vi "NI 5772 (AC) - TIS Mode Enabled (Host)_Independent.vi"() -> ()   [LabVIEW 2020]
doc: "Example Description:\nThis example demonstrates how to enable Time Interleaved Sampling with the NI 5772 adapter module to achieve a sampling rate of 1.6GS/s. This example continuously acquires records of analog input data from the NI 5772 adapter module. It allows you to select an AI channel, trigger type, and record size. This VI must be compiled before it is run. \n\nVI Configuration:\nThis example uses the NI PXI-7952R as the FPGA target by default. If you are using another FPGA target, complete the following steps to configure the host VI to use a VI configured for your FPGA target:\n1. On the block diagram, right-click the Open FPGA VI Reference (NI PXI-7952R) function and select Configure Open FPGA VI Reference.\n2. Browse for a new target by clicking the Browse Project button in the Open VI section.\n3. Select the VI under the target that matches your device. Click OK to select this VI.\n4. Click OK to exit the dialog box and to apply the new selection to the FPGA VI.\n5. Save the VI.\n\nRunning the VI:\n1. Select a RIO Resource that corresponds to the FPGA device configured above.\n2. Clock Configuration: Select the desired clock source for the adapter module.\nAnalog Input: Configure the AI Channel, Record Size, and Trigger Type controls. If you are using the analog trigger type, configure the Trigger Level (V) control.\n3. Click the run arrow to run the VI.\n4. If the Trigger Type is set to Software, click the Software Trigger button to acquire a single record of data. If the Trigger Type is set to Data Edge, a record of data is acquired each time the input signal rises above the trigger level.\n\nThe Record Size, Trigger Type, and Trigger Level (V) controls can all be configured while the VI is running. \n\nNote: The AI Channel control must be configured before the VI is run.\n\nExecution Steps:s\n1. Open a session to the FPGA VI and run the VI.\n2. Wait for the adapter module to load its default configuration.\n3. Configure the NI 5772 for Time Interleaved Sampling (TIS)\n4. The Trigger type and record size for a single record acquisition are configured.\n5. Based on the trigger type, either wait for the software trigger Boolean to assert or configure the desired trigger level and arm the trigger.\n6. After the trigger is armed, a single record of data is acquired and read.\n7. Stop the VI when the stop button is pressed or when an error has occurred. \n8. Close the FPGA VI reference and display any errors."
uses:
  <vilib>/userdefined/High Color/nirio_resource_hc.ctl
  Controls/TIS Mode.ctl
  Controls/FPGA VI Reference.ctl
  <vilib>/FPGAPlugInAG/PXIe-7962R/niLvFpga_Open_PXIe-7962R.vi
  <vilib>/rvi/interface/common/dynamic/niFpgaDynamicAddResources.vi
  <vilib>/Utility/error.llb/Error Cluster From Error Code.vi
  <vilib>/rvi/errors/niLvFpgaAdjustHostInterfaceError.vi
  <vilib>/FPGAPlugInAG/Dynamic/niLvFpga_Close_Dynamic.vi
  <vilib>/rvi/interface/nirviOpenFPGA/nirviOpenFPGA.xnode
  FPGA Bitfiles/acoustoxv3_FPGATarget_NI5772(AC)Digiti_U3W57aODG7w.lvbitx
  <vilib>/rvi/interface/nirviReadWriteControl/nirviReadWriteControl.xnode
  <vilib>/rvi/interface/nirviMethod/nirviMethod.xnode
  <vilib>/rvi/interface/nirviCloseFPGA/nirviCloseFPGA.xnode
  NiFpgaLv.dll
  <vilib>/rvi/interface/Simulation/niFpgaSimulationCallBeginRW.vi
  <vilib>/FPGAPlugInAG/Dynamic/niLvFpga_ReadFifo_Dynamic.vi
  <vilib>/rvi/errors/niLvFpgaMergeErrorWithErrorCode.vi
panel:
  in  "TrigIn_Sim":bool
  in  "TIS Mode":T1=3 items=["TIS Mode (CH0 Only)"=1, "TIS Mode (CH1 Only)"=2, "Dual TIS Mode (CH0 and CH1)"=3]
  out "TIS Configured?":bool
  out "Analog Input":waveform(ext)(graph)={"t0"=timestamp(0 s since 1904-01-01), "dt"=1.25e-09, "Y"=array[2048 elements]} caption="Acquired Waveform"
  out "error out":errorcluster
  in  "stop":bool
  in  "Trigger Level (V)":dbl
  in  "Software Trigger":bool=TRUE
  in  "Record Size":u16=1024
  in  "Trigger Type":enum8{"Software", "Data Edge"}(ring)
  in  "RIO Resource":T2="RIO0"
  out "Configured?":bool
  # "Resource Configuration"
  # "AI Configuration"
  # "For instructions, select Help>>Show Context Help and move the cursor over the VI icon to display help for this VI."
  # "Interleaved Configuration"
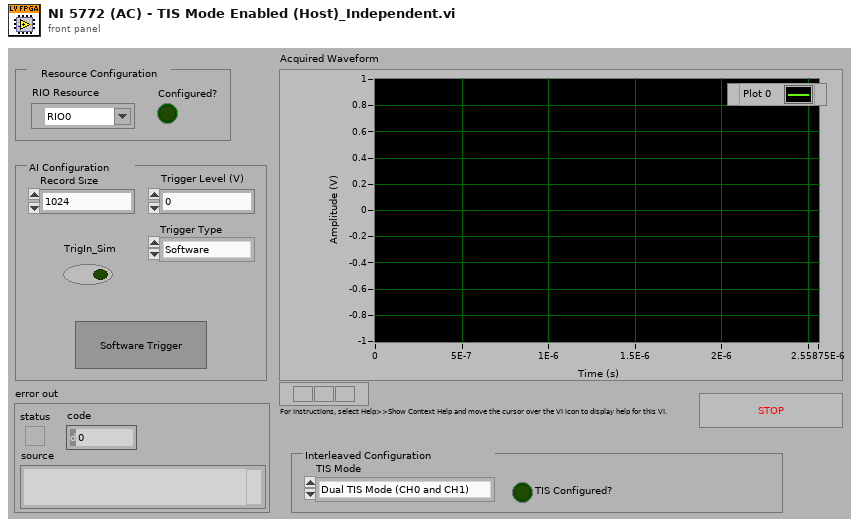
[diagram p1: front panel]
types:
  T1 = typedef "TIS Mode.ctl" = u16
  T2 = typedef "nirio_resource_hc.ctl" = tag
  T3 = typedef "FPGA VI Reference.ctl" = refnum<k20>
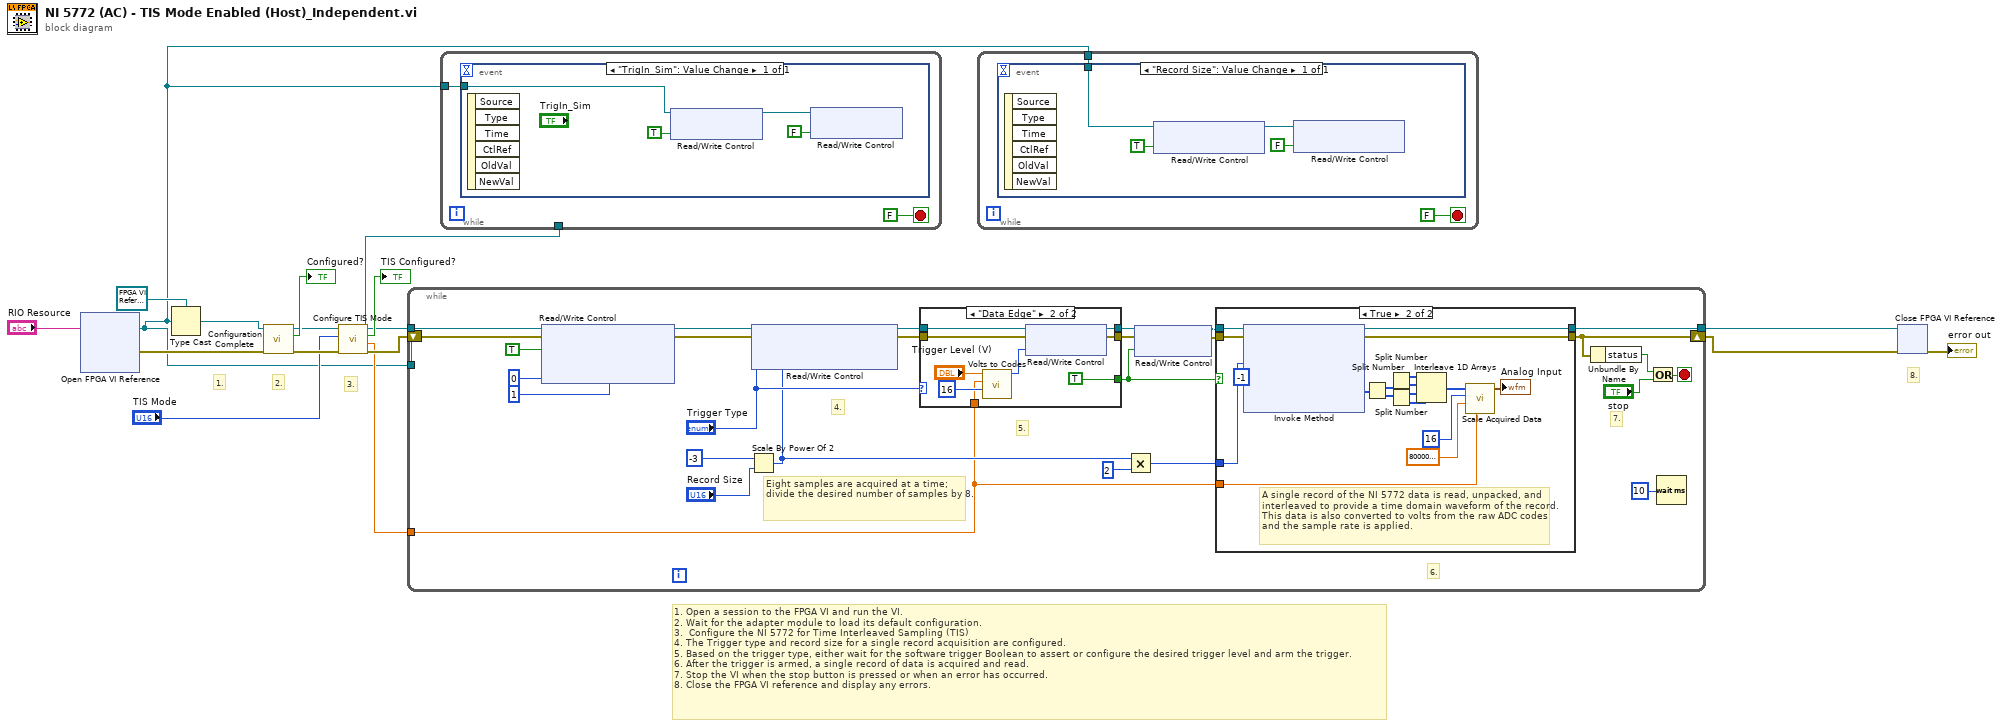
[diagram p0: block diagram]
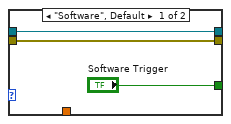
[diagram p3: hidden frame]
diagram:
  # "8."
  # "3."
  # "2."
  # "1."
  # "1. Open a session to the FPGA VI and run the VI.\n2. Wait for the adapter module to load its default configuration.\n3.  Configure the NI 5772 for Time Interleaved Sampling (TIS)\n4. The Trigger type and record size for a single record acquisition are configured.\n5. Based on the trigger type, either wait for the software trigger Boolean to assert or configure the desired trigger level and arm the trigger.\n6. After the trigger is armed, a single record of data is acquired and read.\n7. Stop the VI when the stop button is pressed or when an error has occurred.  \n8. Close the FPGA VI reference and display any errors."
  n1 = xnode "Open FPGA VI Reference"("resource name"="RIO Resource") -> ("FPGA VI Reference Out"=w1:refnum<k20>, "error out"=w14:errorcluster)  [unwired: 1 in]
  n2 = Type Cast(type=T3 refnum ("FPGA VI Reference Out"), x=w1) -> (*(type *) &x=w5:T3)
  n3 = call "Configuration Complete.vi"("error in"=w14, "FPGA VI Reference In"=w5) -> ("error out"=w13:errorcluster, "Configured?"=→"Configured?":bool, "FPGA VI Reference Out"=w11:T3)  [unwired: 7 out]
  n4 = call "Configure TIS Mode.vi"("error in"=w13, "TIS Mode"="TIS Mode", "FPGA VI Reference In"=w11) -> ("error out"=w12:errorcluster, "range (Vpp)"=w7:dbl, "TIS Configured?"=→"TIS Configured?":bool, "FPGA VI Reference Out"=w4:T3)  [unwired: 5 in]
  n5 = while {
    tunnel: [w40] -> w3
    tunnel: w4 -> [_]
    shift-right: [w34] -> w2
    shift-left: w12 -> [w18]
    tunnel: w7 -> [w26]
    tunnel: w1 -> [w20]
    stop <- w31 stop-if-true
    # "7."
    # "Eight samples are acquired at a time; divide the desired number of samples by 8."
    # "6."
    # "5."
    # "4."
    n6 = xnode "Read/Write Control"("FPGA VI Reference In"=w20, "error in"=w18, "vi/nGenTrig"=TRUE, "Delay after Trig [cycles]"=u16 0, "AvgCount"=u16 1) -> ("FPGA VI Reference Out"=w19:refnum<k20>, "error out"=w17:errorcluster)
    n7 = Scale By Power Of 2(n=-3, x="Record Size") -> (x*2^n=w27:u16)
    n8 = xnode "Read/Write Control"("FPGA VI Reference In"=w19, "error in"=w17, "Trigger Type"="Trigger Type", "Quad Samples Per Trigger"=w27) -> ("FPGA VI Reference Out"=w33:refnum<k20>, "error out"=w32:errorcluster)
    n9 = case shown="\"Data Edge\"" "Trigger Type" {
      tunnel: w33 -> [w66 w75]
      tunnel: w32 -> [w65 w74]
      tunnel: [w66 w73] -> w39
      tunnel: [w65 w72] -> w38
      tunnel: ["Software Trigger" TRUE ("Acquire")] -> w35
      tunnel: w26 -> [_ w67]
      frame "Software", Default {
      }
      frame "Data Edge" {
        n10 = call "Volts to Codes.vi"("Number of Bits"=i16 16, "range (Vpp)"=w67, "Data In"="Trigger Level (V)") -> ("Data Out"=w68:i16)  [unwired: 8 out]
        n11 = xnode "Read/Write Control"("FPGA VI Reference In"=w75, "error in"=w74, "Trigger Level"=w68) -> ("FPGA VI Reference Out"=w73:refnum<k20>, "error out"=w72:errorcluster)
      }
    }
    n12 = Multiply(x=w27, y=u16 2) -> (x*y=w25:u16)
    n13 = xnode "Read/Write Control"("FPGA VI Reference In"=w39, "error in"=w38, "Arm Trigger"=w35) -> ("FPGA VI Reference Out"=w37:refnum<k20>, "error out"=w36:errorcluster)
    n14 = case shown="True" w35 {
      tunnel: w37 -> [w44 w63]
      tunnel: w36 -> [w45 w62]
      tunnel: [w45 w61] -> w34
      tunnel: [w44 w60] -> w40
      tunnel: w25 -> [_ w59]
      tunnel: w26 -> [_ w55]
      frame False {
      }
      frame True {
        # "A single record of the NI 5772 data is read, unpacked, and interleaved to provide a time domain waveform of the record. This data is also converted to volts from the raw ADC codes and the sample rate is applied."
        n15 = xnode "Invoke Method"("FPGA VI Reference In"=w63, "error in"=w62, "Number of Elements"=w59, "Timeout (ms)"=-1) -> ("FPGA VI Reference Out"=w60:refnum<k20>, "error out"=w61:errorcluster, "Data"=w54:u64[])  [unwired: 1 out]
        n16 = Split Number(x=w54) -> (hi(x)=w53:u32[], lo(x)=w52:u32[])
        n17 = Split Number(x=w53) -> (hi(x)=w50:u16[], lo(x)=w47:u16[])
        n18 = Split Number(x=w52) -> (hi(x)=w48:u16[], lo(x)=w49:u16[])
        n19 = Interleave 1D Arrays(w50, w47, w48, w49) -> (w51:u16[])
        n20 = call "Scale Acquired Data.vi"("range (V)"=w55, "Sample Rate"=800000000.0, "Number of Bits"=i16 16, "Data In"=w51) -> ("output waveform"=→"Analog Input":waveform(ext))  [unwired: 7 out]
      }
    }
    n21 = Unbundle By Name(w34) -> ("status"=w42:bool)
    n22 = Or(x=w42, y="stop") -> (x .or. y?=w31:bool)
    n23 = Wait (ms)(milliseconds to wait=u32 10) -> ()  [unwired: 1 out]
  }
  n24 = while {
    tunnel: w1 -> [w76]
    tunnel: w4 -> [_]
    stop <- FALSE stop-if-true
    n25 = event shown="[0] \"TrigIn_Sim\": Value Change" {
      selector: _ -> [_]
      dyn-events: _ -> [_]
      timeout: _ -> [_]
      tunnel: w76 -> [w81]
      event "TrigIn_Sim": Value Change {
        n26 = event-data() -> ()  [unwired: 1 in, 6 out]
        n27 = xnode "Read/Write Control"("FPGA VI Reference In"=w81, "TrigIn Simulate"=TRUE ("Arm Trigger")) -> ("FPGA VI Reference Out"=w80:refnum<k20>)  [unwired: 1 in, 1 out]
        n28 = xnode "Read/Write Control"("FPGA VI Reference In"=w80, "TrigIn Simulate"=FALSE ("Arm Trigger")) -> ()  [unwired: 1 in, 2 out]
      }
    }
  }
  n29 = while {
    tunnel: w1 -> [w82]
    stop <- FALSE stop-if-true
    n30 = event shown="[0] \"Record Size\": Value Change" {
      selector: _ -> [_]
      dyn-events: _ -> [_]
      timeout: _ -> [_]
      tunnel: w82 -> [w84]
      event "Record Size": Value Change {
        n31 = event-data() -> ()  [unwired: 1 in, 6 out]
        n32 = xnode "Read/Write Control"("FPGA VI Reference In"=w84, "Clear Accumulator"=TRUE ("Arm Trigger")) -> ("FPGA VI Reference Out"=w85:refnum<k20>)  [unwired: 1 in, 1 out]
        n33 = xnode "Read/Write Control"("FPGA VI Reference In"=w85, "Clear Accumulator"=FALSE ("Arm Trigger")) -> ()  [unwired: 1 in, 2 out]
      }
    }
  }
  n34 = xnode "Close FPGA VI Reference"("FPGA VI Reference In"=w3, "error in"=w2) -> ("error out"=→"error out":errorcluster)
